vi "dfd_Cosine Modulated Synthesis Bank Compute States.vi"(2 "2m":i32, 4 "x":dbl[][](array[numeric])) -> (1 "y":dbl[][](array[numeric]))   [LabVIEW 2017, in "NI_DigFilter_FilterBank.lvlib"]
uses:
  <vilib>/addons/Digital Filter Design/NI_DigFilter_FilterBank.lvlib
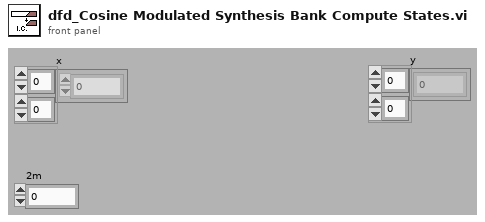
[diagram p1: front panel]
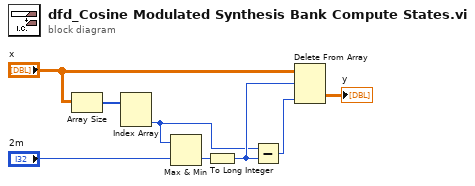
[diagram p0: block diagram]
diagram:
  n1 = Array Size(array="x") -> (size(s)=w2:i32[])
  n2 = Index Array(array=w2) -> (element #2=w3:i32)  [unwired: 2 in, 1 out]
  n3 = Max & Min(x=w3, y="2m") -> (min(x,y)=w4:i32)  [unwired: 1 out]
  n4 = To Long Integer(number=w4) -> (32bit integer=w7:i32)
  n5 = Subtract(x=w3, y=w7) -> (x-y=w5:i32)
  n6 = Delete From Array(array="x", length=w7, index (col)=w5) -> (deleted portion=→"y":dbl[][])  [unwired: 1 in, 1 out]
